vi "ExcelOpenConfigFile.vi"(3 "error in (no error)":errorcluster, 5 "NomProjet":string) -> (0 "sortie d'erreur":errorcluster, 2 "NomProjetOut":string)   [LabVIEW 2017]
uses:
  DefDeType/WhichPath.ctl
panel:
  in  "Excel._Application":refnum<k7>
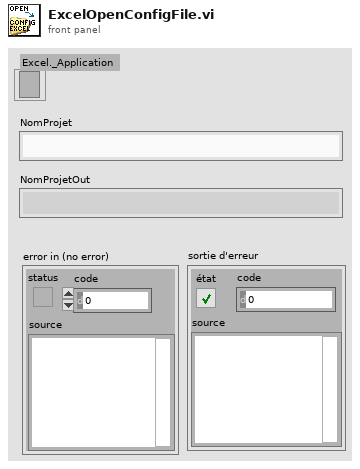
[diagram p1: front panel]
types:
  T1 = typedef "WhichPath.ctl" = enum16{"DossierProjet", "Config", "Meas", "MeasPCI", "MeasCRIO1", "MeasCRIO2", "MeasQualisys", "MeasHBM", "MeasTDMS", "Fig", "Res"}
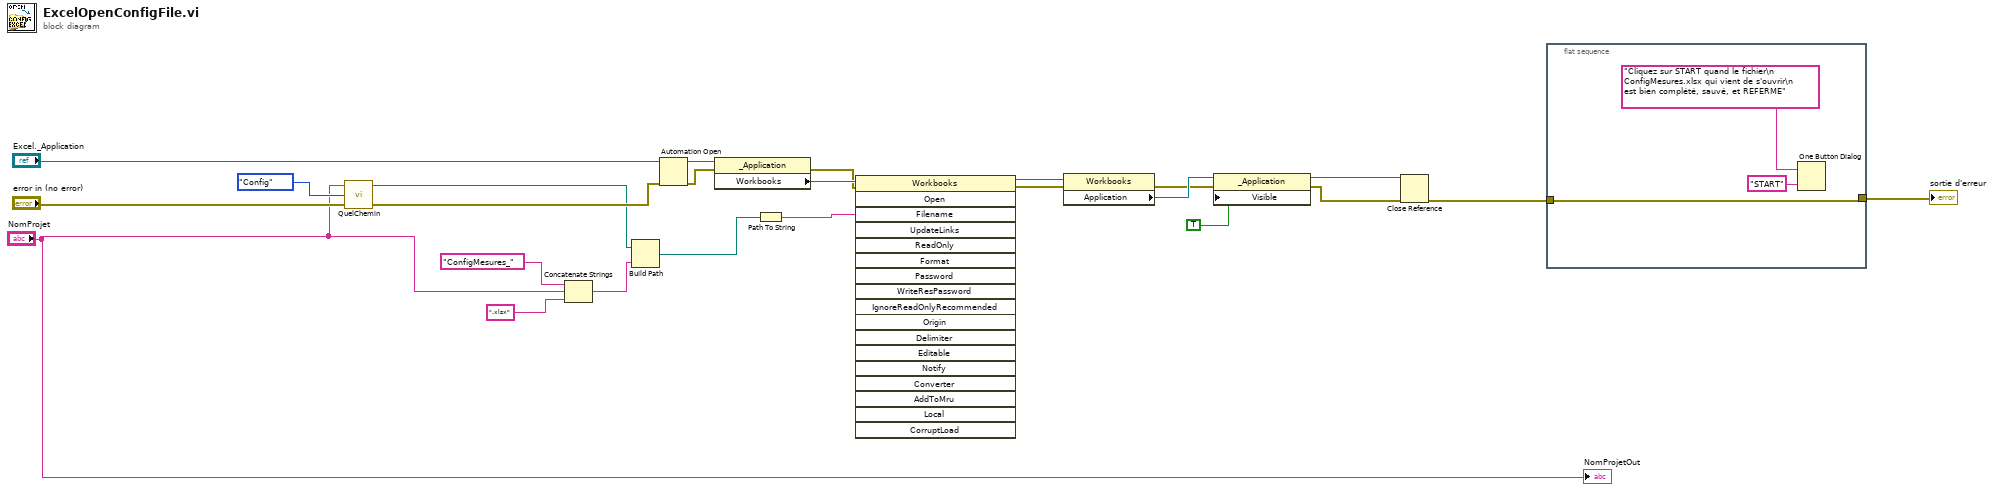
[diagram p0: block diagram]
diagram:
  n1 = call "QuelChemin.vi"("Entrée d'erreur"="error in (no error)", "WhichPath?"=WhichPath."Config", "NomProjet"="NomProjet") -> ("Sortie d'erreur"=w7:errorcluster, "SurDisqueLocal"=w5:path)  [unwired: 1 out]
  n2 = Concatenate Strings("ConfigMesures_" ("nom ou chemin relatif"), "NomProjet", ".xlsx" ("nom ou chemin relatif")) -> (w1:string)
  n3 = Build Path(base path=w5, name or relative path=w1) -> (appended path=w12:path)
  n4 = Automation Open(error in (no error)=w7, Automation Refnum="Excel._Application") -> (Automation Refnum=w24:refnum<k7>, error out=w23:errorcluster)  [unwired: 2 in]
  n5 = property class="_Application"(reference=w24, error in=w23) -> (error out=w21:errorcluster, "Workbooks"=w22:refnum<k7>)  [unwired: 1 out]
  n6 = Path To String(path=w12) -> (string=w20:string)
  n7 = invoke class="Workbooks" method="Open"(reference=w22, error in=w21, "Filename"=w20) -> (reference out=w19:refnum<k7>, error out=w18:errorcluster)  [unwired: 15 in, 16 out]
  n8 = property on="Nœud de propriété" class="Workbooks"(reference=w19, error in=w18) -> (error out=w16:errorcluster, "Application"=w17:refnum<k7>)  [unwired: 1 out]
  n9 = property on="Nœud de propriété" class="_Application"(reference=w17, error in=w16, "Visible"=TRUE) -> (reference out=w15:refnum<k7>, error out=w14:errorcluster)
  n10 = Close Reference(reference=w15, error in (no error)=w14) -> (error out=w10:errorcluster)
  n11 = flat-sequence {
    tunnel: [w27] -> w9
    tunnel: w10 -> [w27]
    frame #0 {
      n12 = One Button Dialog(message="Cliquez sur START quand le fichier\n ConfigMesures.xlsx qui vient de s'ouvrir\n est bien complété, sauvé, et REFERME", button name ("OK")="START" ("nom du bouton (\"OK\")")) -> ()  [unwired: 1 out]
    }
  }
  "sortie d'erreur" <- w9
  "NomProjetOut" <- "NomProjet"
